vi "adam-5000-command-builder.vi"(6 "Output Control":T1, 7 "Current Output State":T1, 8 "chassis slot":u8=1, 9 "ADAM-5000: Chassis ID":u8=1, 11 "Command":T2) -> (1 "trigger write":bool, 3 "Command Out":string, 5 "DO Output":T1)   [LabVIEW 2024]
uses:
  controls/command-enum.ctl
  controls/digital-output-cluster.ctl
panel:
  out "hex integer string":string
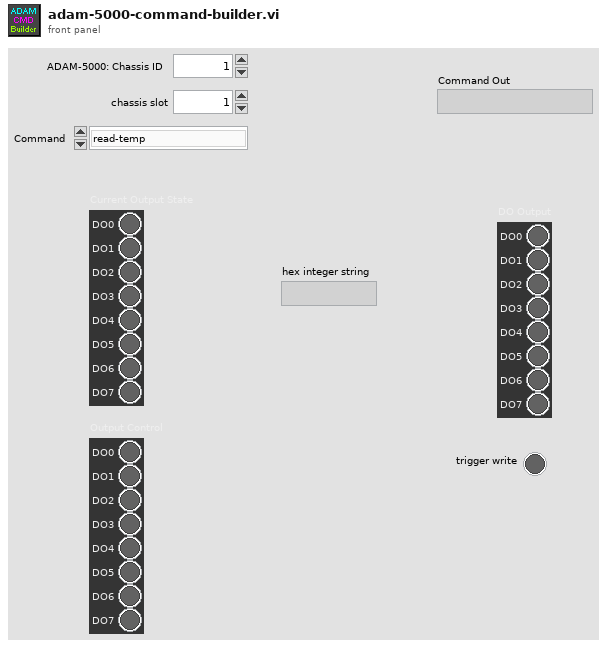
[diagram p1: front panel]
types:
  T1 = typedef "digital-output-cluster.ctl" = cluster{"DO0":bool, "DO1":bool, "DO2":bool, "DO3":bool, "DO4":bool, "DO5":bool, "DO6":bool, "DO7":bool}
  T2 = typedef "command-enum.ctl" = enum16{"read-temp", "read-AI"}
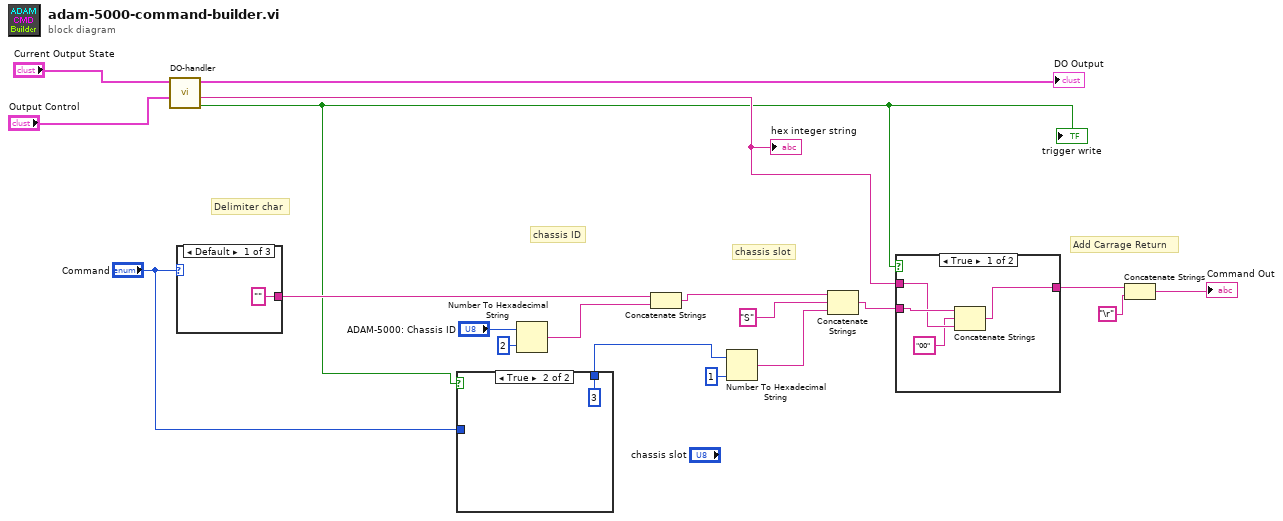
[diagram p0: block diagram]
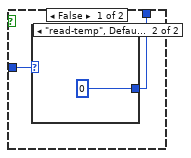
[diagram p2: hidden frame]
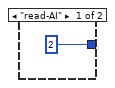
[diagram p3: hidden frame]
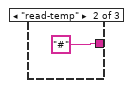
[diagram p5: hidden frame]
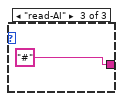
[diagram p6: hidden frame]
diagram:
  # "Add Carrage Return"
  # "chassis slot"
  # "chassis ID"
  # "Delimiter char"
  n1 = call "DO-handler.vi"("Output Control"="Output Control", "Current Output State"="Current Output State") -> ("output state changed"=w1:bool, "hex integer string"=w2:string, "DO Output"=→"DO Output":T1)  [unwired: 5 in, 2 out]
  "trigger write" <- w1
  "hex integer string" <- w2
  n2 = case shown="Default" "Command" {
    tunnel: ["" "#" "#"] -> w10
    frame Default {
    }
    frame "read-temp" {
    }
    frame "read-AI" {
    }
  }
  n3 = case shown="True" w1 {
    tunnel: [w24 u8 3 ("chassis slot")] -> w9
    tunnel: "Command" -> [w23 _]
    frame False {
      n4 = case shown="\"read-temp\", Default" w23 {
        tunnel: [u8 2 ("chassis slot") u8 0 ("chassis slot")] -> w24
        frame "read-AI" {
        }
        frame "read-temp", Default {
        }
      }
    }
    frame True {
    }
  }
  n5 = Number To Hexadecimal String(1:i16 2 ("width (-)"), 2:"ADAM-5000: Chassis ID") -> (0:w11:string)
  n6 = Concatenate Strings(w10, w11) -> (w15:string)
  n7 = Number To Hexadecimal String(1:i16 1 ("width (-)"), 2:w9) -> (0:w17:string)
  n8 = Concatenate Strings(w15, "S" ("string"), w17) -> (w4:string)
  n9 = case shown="True" w1 {
    tunnel: [w30 w32] -> w5
    tunnel: w4 -> [w31 w32]
    tunnel: w2 -> [w29 _]
    frame True {
      n10 = Concatenate Strings(w31, "00" ("string"), w29) -> (w30:string)
    }
    frame False {
    }
  }
  n11 = Concatenate Strings(w5, "\r") -> (→"Command Out":string)
